vi "Plant2_model.vi"(7 "Initial state x(0)":dbl[](array[numeric]), 10 "Input = u(t)":dbl) -> (2 "State = x(t)":dbl[](array[numeric]))   [LabVIEW 2016]
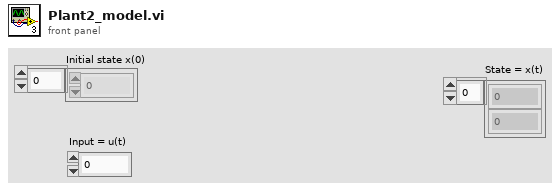
[diagram p1: front panel]
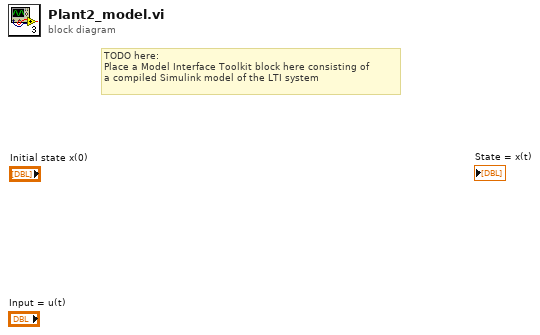
[diagram p0: block diagram]
diagram:
  # "TODO here:\nPlace a Model Interface Toolkit block here consisting of \na compiled Simulink model of the LTI system"
